vi "Puma_GCS_v2.1_UserVersion.vi"(0 "?":refnum<visa-resource-name>="COM3", 1 "?":u32=9600, 9 "XON":u8=17 format="%.0x", 14 "XOFF":u8=19 format="%.0x", 15 "?":u32=10000, 21 "?":bool=TRUE, 24 "?":u8=10 format="%.0x", 25 "bsize":u32=4096) -> ()   [LabVIEW 2015]
doc: "The Advanced Serial Read and Write example performs a Serial Port Read, a Serial Port Write, or a combination of these actions while setting some advanced serial features like buffer size, termination characters, and XON/XOFF flow control. The user selects the actions (read or write) on the front panel. If both are selected, the VI will write the data first, read the data and then close the VISA session that is opened to the port. \n\nThe parameters set for the serial port must match the parameters of the connected instrument or device. In this example, the bytes to read parameter specifies the number of bytes that the serial port reads. If there were more bytes at the port than the number specified in bytes to read, those bytes would not be read. Also, if you specify to read more bytes than the number of bytes actually read, you might receive a timeout error message.\n\nINSTRUCTIONS:\n1) Select the serial resource and configuration parameters (baud rate, data bits, parity, stop bits, flow control).\n2) Termination character can be enabled and set. Also, set the required input buffer size prior to running the example.\n3) Select the operations to be performed. \n4) Connect the serial port to your device. If no device is available, perform a loopback test by doing one of the following. Short pins 2 and 3 on a RS-232 cable or short pin 4 to pin 8 and pin 5 to pin 9 on a RS-485/422 cable. \n5) Run the VI to see the data read. (The \"read string\" will match the \"string to write\" if a loopback test was performed.)\n\nThis example exposes several advanced features that you may need for your application. Not all applications need all the features shown in this example. The input buffer size is likely an important setting that you want to control in your application. This example expands upon the flow control option for XON and XOFF, allowing the user to choose those control characters. The timeout parameter has been brought to the front panel so a user can specify the time period the VISA Read will wait for the number of bytes to read before timing out. Also, the user has several controls for the termination character, which is discussed later.\n\nNote that you can press the write and read buttons and change the bytes to read parameters on the fly, while the example is running. However, you must stop the example to change the other configuration parameters after the example has started running, and then run again.\n\nSet the I/O buffer size slightly higher the amount of data you expect to receive. This is very important for applications that don't use flow control, as you may lose characters if the receive buffer overflows.\n\nSetting the timeout period ensures that the operation returns with a timeout error if the operation cannot be performed in the specified time period. \n\nSome devices require a termination character in order to identify the end of command strings. Some devices send a termination character to signify the end of data to be read. \n\nThis example shows how you can end the Read operation once a termination character is detected in the buffer and/or append a termination character at the end of the Write data. To enable the Read to end on a termination character, use the VISA Configure Serial Port or use the VISA Properties Serial End Mode for Reads, Termination Character Enable, and Termination Character. To end the Write with a termination character, use the VISA Properties Serial End Mode for Writes, the Send End Enable, and Termination Character. In this example, the same termination character is used for both the Read and the Write. You can specify two different characters for your application, if desired.\n\nYour application may require specific characters for the XON/XOFF Flow Control. You can specify these characters with the VISA Properties Flow Control XOFF Character and Flow Control XON Character. Note that if the standard XON and XOFF characters are used, then decimal 17 and 19 are unavailable for data values. Remember that using flow control and setting an adequate buffer size allow you to prevent buffer overflows."
uses:
  <vilib>/Instr/_visa.llb/VISA Configure Serial Port (Instr).vi
panel:
  in  "Fan Shutdown":bool
  in  "DValve / AV6-T":bool
  in  "Flight Control Board":bool
  in  "Safety":bool
  in  "Test Run":bool
  in  "Reset Control":bool
  in  "Primary Safety 2":bool
  out "?":bool
  out "Motors":cluster{dbl, dbl, dbl, dbl}(graph)={1000.0, 1000.0, 1000.0, 1000.0}
  in  "Pressure Transducers":T1(tab)
  out "?":cluster{dbl, dbl, dbl, dbl, dbl}(graph)
  out "?":cluster{dbl, dbl}(graph)
  in  "Thermocouples":T2(tab)
  out "?":cluster{dbl, dbl, dbl, dbl}(graph)
  out "?":cluster{dbl, dbl}(graph)
  out "fo-u":bool
  out "av5-m":bool
  out "fc-u":bool
  out "PT1-U > 4900 PSI":bool
  out "Takeoff Started":bool
  out "Iterations":i32
  out "Reset Triggered":bool
  in  "PixHawk":bool
  in  "XON 2":u8=17 format="%.0x"
  in  "XOFF 2":u8=19 format="%.0x"
  in  "?":bool=TRUE
  in  "bsize 2":u32=4096
  in  "?":u8=10 format="%.0x"
  in  "?":bool=TRUE
  in  "?":u32=10000
  in  "?":refnum<visa-resource-name>="COM3"
  in  "?":u32=9600
  out "Max Values":T3={20.764332288, 0.0, 0.0, 0.0, 0.0, 0.0, 0.0, 201.058, 25.138999999999953, 0.0, 57.16000000000008, 0.0, 8.920000000000016, 15.403999999999996}
  in  "Data Filename":string
  out "Offset 7":dbl=-251.3
  out "Multiplier 7":dbl=1.264
  out "Offset 6":dbl=-250.2
  out "Offset 5":dbl=-250.3
  out "Offset 4":dbl=-1253.0
  out "Offset 3":dbl=-250.9
  out "Offset 2":dbl=-249.8
  out "Offset 1":dbl=-251.0
  out "Multiplier 6":dbl=1.264
  out "Multiplier 5":dbl=1.277
  out "Multiplier 4":dbl=6.36
  out "Multiplier 3":dbl=1.274
  out "Multiplier 2":dbl=1.267
  out "Multiplier 1":dbl=1.277
  in  "Begin Checklist":bool
  out "Manual Abort Tested":bool
  out "Flight Control On":bool
  out "Reset Triggered 2":bool
  out "Primary Safety Active":bool
  out "Craft Triggered Softkill Active":bool
  out "Hardkill Active":bool
  out "ms":dbl=163640.0
  out "vcc 6":bool
  out "gnd 6":bool=TRUE
  out "TCp-2":bool
  out "vcc 5":bool
  out "gnd 5":bool=TRUE
  out "TCp-1":bool
  out "vcc 4":bool
  out "gnd 4":bool=TRUE
  out "TCpw-4":bool
  out "vcc 3":bool
  out "gnd 3":bool=TRUE
  out "TCpw-3":bool
  out "vcc 2":bool
  out "gnd 2":bool=TRUE
  out "TCpw-2":bool
  out "vcc":bool
  out "gnd":bool=TRUE
  out "TCpw-1":bool
  out "Engine 4":dbl=1000.0
  out "Engine 3":dbl=1000.0
  out "Engine 2":dbl=1000.0
  out "Engine 1":dbl=1000.0
  out "soft kill ind":bool
  out "dump fuel ind":bool
  out "abort ind":bool
  out "run ind":bool
  out "av6-t ind":bool
  out "Control input":bool
  out "return":bool
  out "Control (on/off)":bool
  out "PT5-M":dbl=-6.084000000000003
  out "PT2-M":dbl=-10.039999999999992
  out "PT2-U":dbl=-250.3
  out "PT1-U":dbl=-38.24000000000001
  out "PT3-M":dbl=-141.336
  out "PT1-M":dbl=9.934999999999945
  out "PT4-M":dbl=181.90299999999996
  out "TCp-2":dbl=-2.0
  out "TCp-1":dbl=-2.0
  out "TCpw-4":dbl=-2.0
  out "TCpw-3":dbl=-2.0
  out "TCpw-2":dbl=-2.0
  out "TCpw-1":dbl=-2.0
  out "Output":string="h:;"
  in  "?":enum32{"Test"}(tab)
  in  "Primary Safety":bool=TRUE
  in  "Soft Kill":bool
  in  "Simulate":bool
  in  "Reset FC":bool
  in  "Full Power":bool
  in  "Secondary Safety":bool=TRUE
  in  "Takeoff":bool
  in  "Calibrate":bool
  in  "Profile Selector":u16 max=9 step=1
  in  "abort":bool
  out "?":dbl(graph)=20.40794784
  in  "Send":bool=TRUE
  in  "Recieve":bool=TRUE
  in  "bytes to read 2":u32=1000
  out "?":u32=107
  out "?":string[](array[string])=["339", "205", "86", "191", "0", "190", "194", "-2.00", "-2.00", "-2.00", "-2.00", "-2.00", "-2.00", "555", "1000", "1000", "1000", "1000", "163640"]
  out "?":string[](array[string])=["p:339,205,86,191,0,190,194", "t:-2.00,-2.00,-2.00,-2.00,-2.00,-2.00", "v:555", "m:1000,1000,1000,1000", "h:", "s:163640", ""]
  out "Voltage Sensor":dbl=20.40794784
  in  "dump fuel":bool
  in  "?":enum32{"Ignore"}(tab)
  out "?":bool=TRUE
  out "String":string
  in  "String 3":string
  in  "?":bool=TRUE
  in  "tank iso":bool
  in  "Av-6Tt":bool
  in  "FC-U Toggle":bool
  in  "FOU":bool
  out "?":dbl(slide) scale=0.2..200.0
  out "FO-U":bool
  out "FC-U":bool
  out "AV6-T":bool
  out "AV1-T":bool
  out "AV3-T":bool
  out "AV4-T":bool
  out "AV5-T":bool
  out "AV2-T":bool
  # "Data From Craft:"
  # "FO-U"
  # "FC-U"
  # "receive"
  # "send"
  # "AV6-M"
  # "AV5-M"
  # "AV1-M"
  # "AV2-M"
  # "AV3-M"
  # "AV4-M"
  # "green=open - check thermocouple attachments\nred=short gnd - contact Power or GNC\nblue=short vcc - contact Power or GNC"
  # "Voltage"
  # "TCp2-M"
  # "Tcw1-E"
  # "TCp1-M"
  # "TCw4-E"
  # "TCw3-E"
  # "TCw2-E"
  # "PT4-M"
  # "PT1-M"
  # "PT3-M"
  # "PT1-U"
  # "PT2-U"
  # "PT2-M"
  # "PT5-M"
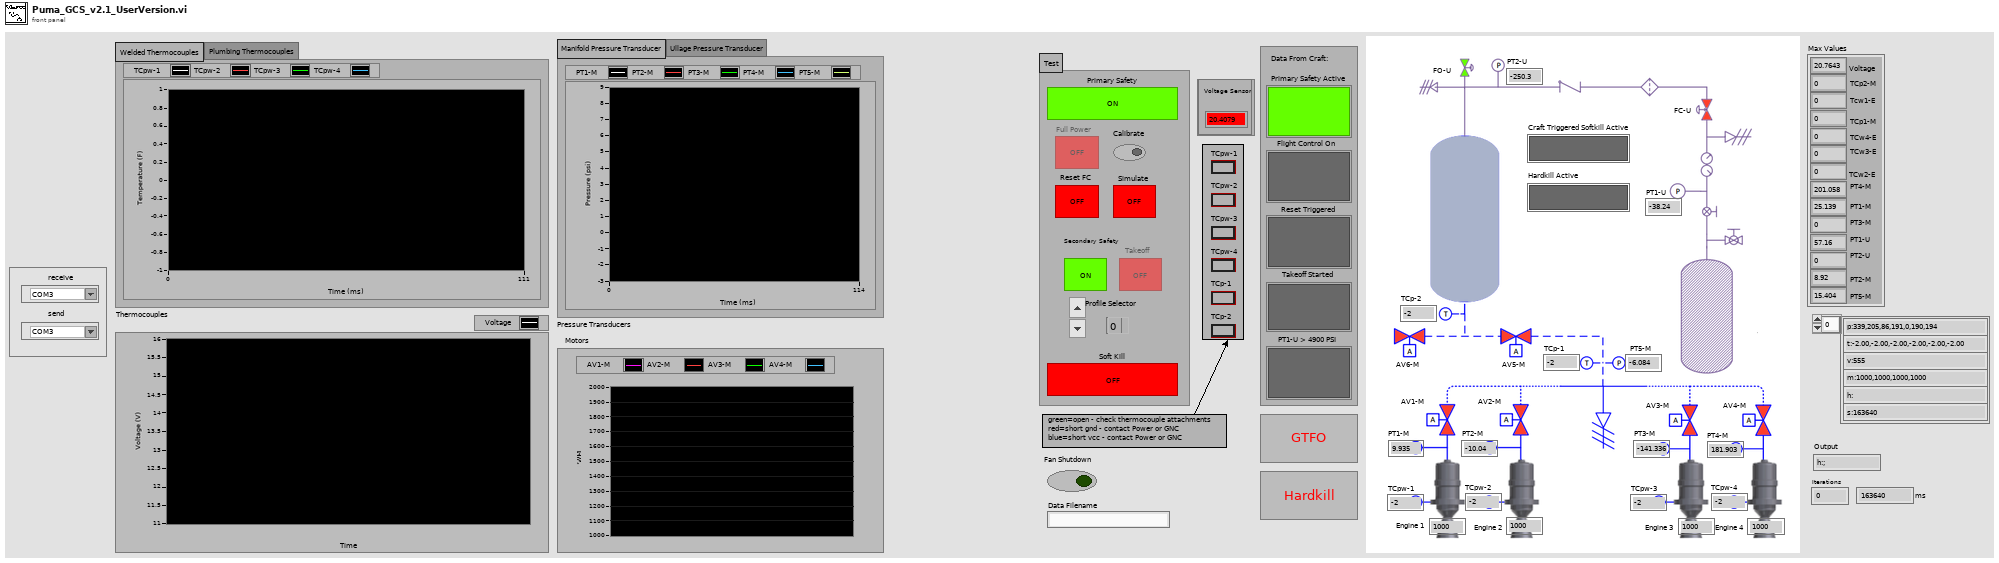
[diagram p1: front panel]
types:
  T1 = enum32{"Manifold Pressure Transducer", "Ullage Pressure Transducer"}
  T2 = enum32{"Welded Thermocouples", "Plumbing Thermocouples"}
  T3 = cluster{dbl, dbl, dbl, dbl, dbl, dbl, dbl, dbl, dbl, dbl, dbl, dbl, dbl, dbl}
  T4 = enum16{"open", "replace", "create", "open or create", "replace or create", "replace or create with confirmation"}
  T5 = cluster{"Output":dbl, dbl, dbl, dbl, dbl, dbl, dbl, "Output":dbl, "Output":dbl, "Output":dbl, "Output":dbl, "Output":dbl, "Output":dbl, "Output":dbl}
  T6 = cluster{"Output":dbl, "Output":dbl, "Output":dbl, "Output":dbl, "Output":dbl}
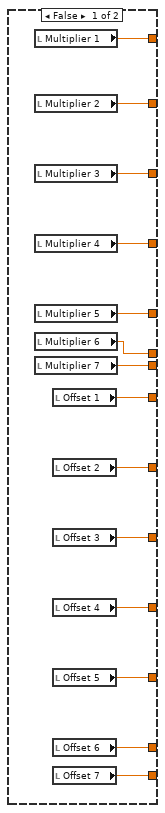
[diagram p3: hidden frame]
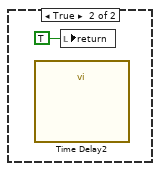
[diagram p13: hidden frame]
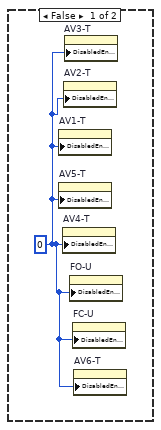
[diagram p16: hidden frame]
diagram:
  w2 = TRUE
  w1 = FALSE
  w51 = u16 16  # I/O Receive Buffer mask
  w75 = u16 16  # I/O Receive Buffer mask
  # "Comment"
  # "Set default values"
  n1 = while {
    stop <- FALSE stop-if-true
    n2 = case shown="True" "Calibrate" {
      tunnel: [w109 w123] -> w93
      tunnel: [w108 w122] -> w92
      tunnel: [w107 w121] -> w91
      tunnel: [w106 w120] -> w90
      tunnel: [w105 w119] -> w89
      tunnel: [w104 w118] -> w88
      tunnel: [w103 w117] -> w87
      tunnel: [w101 w116] -> w86
      tunnel: [w102 w115] -> w85
      tunnel: [w100 w114] -> w84
      tunnel: [w99 w113] -> w83
      tunnel: [w98 w112] -> w82
      tunnel: [w97 w111] -> w81
      tunnel: [w96 w110] -> w80
      frame False {
        n3 = local read "Multiplier 1"() -> (w109:dbl)
        n4 = local read "Multiplier 2"() -> (w108:dbl)
        n5 = local read "Multiplier 3"() -> (w107:dbl)
        n6 = local read "Multiplier 4"() -> (w106:dbl)
        n7 = local read "Multiplier 5"() -> (w105:dbl)
        n8 = local read "Multiplier 6"() -> (w104:dbl)
        n9 = local read "Multiplier 7"() -> (w103:dbl)
        n10 = local read "Offset 1"() -> (w101:dbl)
        n11 = local read "Offset 2"() -> (w102:dbl)
        n12 = local read "Offset 3"() -> (w100:dbl)
        n13 = local read "Offset 4"() -> (w99:dbl)
        n14 = local read "Offset 5"() -> (w98:dbl)
        n15 = local read "Offset 6"() -> (w97:dbl)
        n16 = local read "Offset 7"() -> (w96:dbl)
      }
      frame True {
        n17 = call "P configure.vi"() -> ("Multiplier 1"=w123:dbl, "Offset 1"=w116:dbl, "Multiplier 2"=w122:dbl, "Offset 2"=w115:dbl, "Multiplier 3"=w121:dbl, "Offset 6"=w111:dbl, "Offset 3"=w114:dbl, "Offset 7"=w110:dbl, "Multiplier 4"=w120:dbl, "Multiplier 7"=w117:dbl, "Multiplier 6"=w118:dbl, "Offset 5"=w112:dbl, "Multiplier 5"=w119:dbl, "Offset 4"=w113:dbl)  [unwired: 2 in]
      }
    }
    "Multiplier 1" <- w93
    "Multiplier 2" <- w92
    "Multiplier 3" <- w91
    "Multiplier 4" <- w90
    "Multiplier 5" <- w89
    "Offset 1" <- w86
    "Offset 2" <- w85
    "Offset 3" <- w84
    "Offset 4" <- w83
    "Offset 5" <- w82
    "Offset 6" <- w81
    "Multiplier 7" <- w87
    "Offset 7" <- w80
    "Multiplier 6" <- w88
  }
  n18 = while {
    stop <- FALSE stop-if-true
    n19 = local read "Control (on/off)"() -> (w124:bool)
    n20 = Wait Until Next ms Multiple(millisecond multiple=50) -> ()  [unwired: 1 out]
    n21 = case shown="True" w124 {
      frame False {
      }
      frame True {
        n22 = local read "dump fuel ind"() -> (w142:bool)
        n23 = local read "soft kill ind"() -> (w140:bool)
        n24 = local read "av6-t ind"() -> (w143:bool)
        n25 = local read "abort ind"() -> (w144:bool)
        n26 = local read "fc-u"() -> (w130:bool)
        n27 = local read "av5-m"() -> (w132:bool)
        n28 = local read "fo-u"() -> (w134:bool)
        n29 = local read "run ind"() -> (w141:bool)
        n30 = case shown="True" w140 {
          tunnel: [_ "Are you sure you want to Softkill?"] -> w135
          frame False {
          }
          frame True {
          }
        }
        n31 = case shown="True" w142 {
          tunnel: [_ "Are you sure you want to Dump Fuel?"] -> w137
          frame False {
          }
          frame True {
          }
        }
        n32 = case shown="True" w143 {
          tunnel: [_ "Are you sure you want to Open AV6-M?"] -> w138
          frame False {
          }
          frame True {
          }
        }
        n33 = case shown="True" w144 {
          tunnel: [_ "Are you sure you want to Abort?"] -> w139
          frame False {
          }
          frame True {
          }
        }
        n34 = case shown="True" w134 {
          tunnel: [_ "Are you sure you want to close FO-U?"] -> w133
          frame False {
          }
          frame True {
          }
        }
        n35 = case shown="True" w130 {
          tunnel: [_ "Are you sure you want to open FC-U?"] -> w129
          frame False {
          }
          frame True {
          }
        }
        n36 = case shown="True" w132 {
          tunnel: [_ "Are you sure you want to open AV5-M?"] -> w131
          frame False {
          }
          frame True {
          }
        }
        n37 = case shown="True" w141 {
          tunnel: [_ "Are you sure you want to Run?"] -> w136
          frame False {
          }
          frame True {
          }
        }
        n38 = Concatenate Strings(w135, w136, w137, w138, w139, w133, w131, w129) -> (w128:string)
        n39 = call "DialogBoxSubVI.vi"("Prompt"=w128) -> ("Boolean"=w127:bool)  [unwired: 9 in]
        n40 = case shown="False" w127 {
          frame False {
            n41 = call "Time Delay"() -> ()  [unwired: 11 in, 1 out]
            n42 = local write "return"(TRUE) -> ()
          }
          frame True {
            n43 = call "Time Delay2"() -> ()  [unwired: 11 in, 1 out]
            n44 = local write "return"(TRUE) -> ()
          }
        }
        n45 = local write "Control input"(w127) -> ()
      }
    }
  }
  n46 = call-poly "VISA Configure Serial Port"("VISA resource name"="?", "timeout (10sec)"="?", "termination char\n(0xA = '\\n' = LF)"="?", "Enable Termination\nChar (T)"="?", "baud rate (9600)"="?") -> ("VISA resource name out"=w64:refnum<visa-resource-name>, "error out"=w67:errorcluster)  [unwired: 5 in, 4 out]
  n47 = call-poly "VISA Configure Serial Port"("VISA resource name"="?", "timeout (10sec)"="?", "termination char\n(0xA = '\\n' = LF)"="?", "Enable Termination\nChar (T)"="?", "baud rate (9600)"="?") -> ("VISA resource name out"=w40:refnum<visa-resource-name>, "error out"=w43:errorcluster)  [unwired: 5 in, 4 out]
  n48 = case shown="True" "?" {
    selector: "?" -> [_ w157]
    tunnel: w64 -> [w155 w163]
    tunnel: w67 -> [w156 w162]
    tunnel: [w155 w161] -> w65
    tunnel: [w156 w160] -> w66
    tunnel: "?" -> [_ w158]
    frame False {
    }
    frame True {
      w159 = u16 2 items=["None", "LastBit", "TermChar", "Break"] ("Serial Settings:Serial End Mode for Writes")
      n49 = property class="Instr"(reference=w163, error in=w162, "Serial Settings:End Mode for Writes"=w159, "Message Based Settings:Send End Enable"=w157, "Message Based Settings:Termination Character"=w158) -> (reference out=w161:refnum<visa-resource-name>, error out=w160:errorcluster)
    }
  }
  n50 = case shown="True" "?" {
    selector: "?" -> [_ w166]
    tunnel: w40 -> [w164 w172]
    tunnel: w43 -> [w165 w171]
    tunnel: [w164 w170] -> w41
    tunnel: [w165 w169] -> w42
    tunnel: "?" -> [_ w167]
    frame False {
    }
    frame True {
      w168 = u16 2 items=["None", "LastBit", "TermChar", "Break"] ("Serial Settings:Serial End Mode for Writes")
      n51 = property class="Instr"(reference=w172, error in=w171, "Serial Settings:End Mode for Writes"=w168, "Message Based Settings:Send End Enable"=w166, "Message Based Settings:Termination Character"=w167) -> (reference out=w170:refnum<visa-resource-name>, error out=w169:errorcluster)
    }
  }
  n52 = property on="Secondary Safety" class="Bool (strict)"("Value"=w2) -> ()  [unwired: 2 in, 2 out]
  n53 = property on="Primary Safety" class="Bool (strict)"("Value"=w2) -> ()  [unwired: 2 in, 2 out]
  n54 = property on="Reset FC" class="Bool (strict)"("Value"=w1) -> ()  [unwired: 2 in, 2 out]
  n55 = property on="Simulate" class="Bool (strict)"("Value"=w1) -> ()  [unwired: 2 in, 2 out]
  n56 = property on="Craft Triggered Softkill Active" class="Bool (strict)"("Value"=w1) -> ()  [unwired: 2 in, 2 out]
  n57 = property on="Hardkill Active" class="Bool (strict)"("Value"=w1) -> ()  [unwired: 2 in, 2 out]
  n58 = property on="Takeoff Started" class="Bool (strict)"("Value"=w1) -> ()  [unwired: 2 in, 2 out]
  n59 = property on="FOU" class="Bool (strict)"("Value"=w1) -> ()  [unwired: 2 in, 2 out]
  n60 = property on="Soft Kill" class="Bool (strict)"("Value"=w1) -> ()  [unwired: 2 in, 2 out]
  n61 = property on="dump fuel" class="Bool (strict)"("Value"=w1) -> ()  [unwired: 2 in, 2 out]
  n62 = property on="abort" class="Bool (strict)"("Value"=w1) -> ()  [unwired: 2 in, 2 out]
  n63 = property on="Manual Abort Tested" class="Bool (strict)"("Value"=w1) -> ()  [unwired: 2 in, 2 out]
  n64 = Build Path(base path=path "C:/Users/Lunar Lion/Desktop/Puma_Test_Data" ("file path (use dialog)"), name or relative path="Data Filename") -> (appended path=w59:path)
  n65 = Build Array("PT4-M_a", "PT1-M_a", "PT3-M_a", "PT1-U_a", "PT2-U_a", "PT2-M_a", "PT5-M_a", "PT4-M", "PT1-M", "PT3-M", "PT1-U", "PT2-U", "PT2-M", "PT5-M", "TCp2-M", "TCw1-E", "TCp1-M", "TCw4-E", "TCw3-E", "TCw2-E", "Voltage", "Motor1", "Motor2", "Motor3", "Motor4", "Statestring") -> (w12:string[])
  n66 = VISA Set I/O Buffer Size(VISA resource name=w65, mask (16)=w75, size (4096)="bsize", error in (no error)=w66) -> (VISA resource name out=w71:refnum<visa-resource-name>, error out=w70:errorcluster)
  n67 = VISA Set I/O Buffer Size(VISA resource name=w41, mask (16)=w51, size (4096)="bsize 2", error in (no error)=w42) -> (VISA resource name out=w47:refnum<visa-resource-name>, error out=w46:errorcluster)
  n68 = Open/Create/Replace File(file path (use dialog)=w59, operation (0:open)=T4."replace or create with confirmation") -> (refnum out=w9:refnum<file>)  [unwired: 4 in, 2 out]
  n69 = Array To Spreadsheet String(array=w12, 3:"%s" ("format string")) -> (spreadsheet string=w10:string)  [unwired: 1 in]
  n70 = property class="Instr"(reference=w71, error in=w70, "Serial Settings:Flow Control XON Character"="XON", "Serial Settings:Flow Control XOFF Character"="XOFF") -> (reference out=w63:refnum<visa-resource-name>, error out=w62:errorcluster)
  n71 = property class="Instr"(reference=w47, error in=w46, "Serial Settings:Flow Control XON Character"="XON 2", "Serial Settings:Flow Control XOFF Character"="XOFF 2") -> (reference out=w39:refnum<visa-resource-name>)  [unwired: 1 out]
  n72 = Write to Text File(file (use dialog)=w9, text=w10) -> (refnum out=w8:refnum<file>)  [unwired: 2 in, 2 out]
  n73 = while {
    tunnel: w63 -> [w338]
    tunnel: w62 -> [w406]
    tunnel: [w322] -> w7
    tunnel: [w321] -> w61
    shift-right: [w506] -> _
    shift-left: _ -> [w505]
    shift-right: [w231] -> _
    shift-left: _ -> [w467]
    shift-right: [w475] -> _
    shift-left: _ -> [w476]
    shift-right: [w466] -> _
    shift-left: _ -> [w490]
    shift-right: [w249] -> _
    shift-left: _ -> [w488]
    shift-right: [w468] -> _
    shift-left: _ -> [w471]
    shift-right: ["Begin Checklist"] -> _
    shift-left: _ -> [w387]
    tunnel: w8 -> [w359]
    tunnel: [w356] -> w58
    shift-right: [w341] -> _
    shift-left: T3 {0.0, 0.0, 0.0, 0.0, 0.0, 0.0, 0.0, 0.0, 0.0, 0.0, 0.0, 0.0, 0.0, 0.0} -> [w340]
    tunnel: w39 -> [_]
    shift-right: [w245] -> _
    shift-left: _ -> [w248]
    shift-right: [w242] -> _
    shift-left: _ -> [w243]
    shift-right: [w239] -> _
    shift-left: _ -> [w240]
    i -> [w326]
    stop <- FALSE stop-if-true
    w193 = 140.0
    w195 = 1400.0
    w200 = 900.0
    w270 = u32 13816530
    w272 = 120.0
    w275 = 1200.0
    w271 = u32 16776704
    w281 = 800.0
    # "e"
    # "The purpose of this indicator is not entirely clear"
    # "Hidden test run button."
    # "Hidden secondary safety."
    # "Hidden reset control button."
    # "Hidden flight control board button."
    # "Un-named indicator, hidden."
    # "Hidden dump valve indicator/button?"
    # "Hidden primary safety"
    # "Tabs for the main command buttons."
    # "Ignore tab with the two strings and indicator light."
    # "Above nominal thresholds:\n   All PTs except PT1-U: 800\n   TCpw-1 to 4: 1200\n   TCp-1 and 2: 120"
    # "The second String \nParsing Indicator"
    # "String Parsing Indicator control"
    # "ENSURE THE PTs ARE HOOKED UP PROPERLY"
    # "Here, if PT1-U indicates a pressure greater than 5000 psi,\nthe indicator represented in the case structure is turned green. Otherwise, it is turned red."
    # "AV6 -T Case"
    # "AV5-T Case"
    # "AV5-T Toggle"
    n74 = case shown="True" FALSE {
      frame False {
      }
      frame True {
        w678 = FALSE
        n75 = local write "FOU"(TRUE) -> ()
        n76 = local write "AV1-T"(w678) -> ()
        n77 = local write "AV2-T"(w678) -> ()
        n78 = local write "AV3-T"(w678) -> ()
        n79 = local write "AV4-T"(w678) -> ()
        n80 = local write "FC-U Toggle"(w678) -> ()
        n81 = local write "tank iso"(w678) -> ()
      }
    }
    n82 = property on="abort" class="Bool (strict)"() -> ("Value"=w302:bool)  [unwired: 2 in, 2 out]
    n83 = local read "Voltage Sensor"() -> (w234:dbl)
    n84 = case shown="False" w302 {
      frame False {
        n85 = property on="Soft Kill" class="Bool (strict)"() -> ("Value"=w661:bool)  [unwired: 2 in, 2 out]
        n86 = case shown="True" w661 {
          frame False {
            n87 = property on="dump fuel" class="Bool (strict)"("DisabledEnum"=0) -> ()  [unwired: 2 in, 2 out]
          }
          frame True {
            n88 = property on="dump fuel" class="Bool (strict)"("DisabledEnum"=2) -> ()  [unwired: 2 in, 2 out]
          }
        }
      }
      frame True {
        n89 = property on="dump fuel" class="Bool (strict)"("DisabledEnum"=2) -> ()  [unwired: 2 in, 2 out]
      }
    }
    n90 = Greater?(x=w234, y=14.5) -> (0:w237:bool)
    n91 = Less Or Equal?(x=w234, y=16.8) -> (x <= y?=w317:bool)
    n92 = Less Or Equal?(x=w234, y=15.5) -> (x <= y?=w312:bool)
    n93 = Greater?(x=w234, y=15.5) -> (0:w316:bool)
    n94 = Greater?(x=w234, y=16.8) -> (0:w309:bool)
    n95 = Less Or Equal?(x=w234, y=17.0) -> (x <= y?=w310:bool)
    n96 = Greater?(x=w234, y=17.0) -> (0:w305:bool)
    n97 = And(x=w309, y=w310) -> (x .and. y?=w308:bool)
    n98 = And(x=w237, y=w312) -> (x .and. y?=w313:bool)
    n99 = And(x=w316, y=w317) -> (x .and. y?=w318:bool)
    n100 = Less Or Equal?(x=w234, y=14.5) -> (x <= y?=w235:bool)
    n101 = case shown="True" w313 {
      frame False {
      }
      frame True {
        n102 = property on="Voltage Sensor" class="DigNum (strict)"("NumText.TextColor"=u32 0) -> ()  [unwired: 2 in, 2 out]
        n103 = property on="Voltage Sensor" class="DigNum (strict)"("NumText.BGColor"=u32 16776704) -> ()  [unwired: 2 in, 2 out]
      }
    }
    n104 = case shown="True" w235 {
      frame False {
      }
      frame True {
        n105 = property on="Voltage Sensor" class="DigNum (strict)"("NumText.BG Color"=u32 16711680) -> ()  [unwired: 2 in, 2 out]
      }
    }
    n106 = case shown="True" w318 {
      frame False {
      }
      frame True {
        n107 = property on="Voltage Sensor" class="DigNum (strict)"("NumText.BGColor"=u32 6618880) -> ()  [unwired: 2 in, 2 out]
        n108 = property on="Voltage Sensor" class="DigNum (strict)"("NumText.TextColor"=u32 16777222) -> ()  [unwired: 2 in, 2 out]
      }
    }
    n109 = case shown="True" w308 {
      frame False {
      }
      frame True {
        n110 = property on="Voltage Sensor" class="DigNum (strict)"("NumText.BGColor"=u32 16776704) -> ()  [unwired: 2 in, 2 out]
        n111 = property on="Voltage Sensor" class="DigNum (strict)"("NumText.TextColor"=u32 16777222) -> ()  [unwired: 2 in, 2 out]
      }
    }
    n112 = case shown="True" w305 {
      frame False {
      }
      frame True {
        n113 = property on="Voltage Sensor" class="DigNum (strict)"("NumText.BGColor"=u32 16711704) -> ()  [unwired: 2 in, 2 out]
      }
    }
    n114 = Exclusive Or(1:w490, 2:"abort") -> (0:w492:bool)
    n115 = property on="TCpw-1" class="DigNum (strict)"() -> ("Value"=w196:dbl)  [unwired: 2 in, 2 out]
    n116 = property on="TCpw-2" class="DigNum (strict)"() -> ("Value"=w197:dbl)  [unwired: 2 in, 2 out]
    n117 = property on="TCpw-3" class="DigNum (strict)"() -> ("Value"=w198:dbl)  [unwired: 2 in, 2 out]
    n118 = property on="TCpw-4" class="DigNum (strict)"() -> ("Value"=w199:dbl)  [unwired: 2 in, 2 out]
    n119 = case shown="True" w492 {
      tunnel: [w742 w744] -> w466
      tunnel: w490 -> [w742 w743]
      frame False {
      }
      frame True {
        n120 = case shown="False" w743 {
          tunnel: [w745 FALSE ("T button?")] -> w744
          frame False {
            w746 = TRUE
            n121 = local write "abort ind"(w746) -> ()
            n122 = local write "Control (on/off)"(w746) -> ()
            n123 = local read "Control input"() -> (w745:bool)
          }
          frame True {
          }
        }
      }
    }
    n124 = Exclusive Or(1:w471, 2:"Soft Kill") -> (0:w469:bool)
    n125 = property on="TCp-2" class="DigNum (strict)"() -> ("Value"=w192:dbl)  [unwired: 2 in, 2 out]
    n126 = property on="TCp-1" class="DigNum (strict)"() -> ("Value"=w194:dbl)  [unwired: 2 in, 2 out]
    n127 = property on="PT2-M" class="DigNum (strict)"() -> ("Value"=w201:dbl)  [unwired: 2 in, 2 out]
    n128 = property on="PT1-M" class="DigNum (strict)"() -> ("Value"=w202:dbl)  [unwired: 2 in, 2 out]
    n129 = property on="PT3-M" class="DigNum (strict)"() -> ("Value"=w203:dbl)  [unwired: 2 in, 2 out]
    n130 = property on="PT4-M" class="DigNum (strict)"() -> ("Value"=w204:dbl)  [unwired: 2 in, 2 out]
    n131 = property on="PT5-M" class="DigNum (strict)"() -> ("Value"=w205:dbl)  [unwired: 2 in, 2 out]
    n132 = property on="PT2-U" class="DigNum (strict)"() -> ("Value"=w206:dbl)  [unwired: 2 in, 2 out]
    n133 = Exclusive Or(1:w488, 2:"dump fuel") -> (0:w489:bool)
    n134 = case shown="True" w469 {
      tunnel: [w732 w734] -> w468
      tunnel: w471 -> [w732 w733]
      frame False {
      }
      frame True {
        n135 = case shown="False" w733 {
          tunnel: [w735 _] -> w734
          frame False {
            w736 = TRUE
            n136 = local write "soft kill ind"(w736) -> ()
            n137 = local write "Control (on/off)"(w736) -> ()
            n138 = local read "Control input"() -> (w735:bool)
          }
          frame True {
          }
        }
      }
    }
    n139 = Greater Or Equal?(x=w192, y=w272) -> (x >= y?=w273:bool)
    n140 = Greater Or Equal?(x=w194, y=w272) -> (x >= y?=w274:bool)
    n141 = Greater Or Equal?(x=w196, y=w275) -> (x >= y?=w279:bool)
    n142 = Greater Or Equal?(x=w197, y=w275) -> (x >= y?=w278:bool)
    n143 = Greater Or Equal?(x=w198, y=w275) -> (x >= y?=w277:bool)
    n144 = Greater Or Equal?(x=w199, y=w275) -> (x >= y?=w276:bool)
    n145 = Greater Or Equal?(x=w201, y=w281) -> (x >= y?=w285:bool)
    n146 = Greater Or Equal?(x=w202, y=w281) -> (x >= y?=w286:bool)
    n147 = Greater Or Equal?(x=w203, y=w281) -> (x >= y?=w284:bool)
    n148 = Greater Or Equal?(x=w204, y=w281) -> (x >= y?=w283:bool)
    n149 = Greater Or Equal?(x=w205, y=w281) -> (x >= y?=w282:bool)
    n150 = Greater Or Equal?(x=w206, y=w281) -> (x >= y?=w280:bool)
    n151 = case shown="True" w489 {
      tunnel: [w737 w739] -> w249
      tunnel: w488 -> [w737 w738]
      frame False {
      }
      frame True {
        n152 = case shown="False" w738 {
          tunnel: [w741 _] -> w739
          frame False {
            w740 = TRUE
            n153 = local write "Control (on/off)"(w740) -> ()
            n154 = local write "dump fuel ind"(w740) -> ()
            n155 = local read "Control input"() -> (w741:bool)
          }
          frame True {
          }
        }
      }
    }
    n156 = case shown="True" w273 {
      tunnel: w271 -> [_ w593]
      tunnel: w270 -> [w589 _]
      tunnel: w193 -> [_ w591]
      tunnel: w192 -> [_ w590]
      frame False {
        n157 = property on="TCp-2" class="DigNum (strict)"("NumText.BGColor"=w589) -> ()  [unwired: 2 in, 2 out]
      }
      frame True {
        n158 = Greater Or Equal?(x=w590, y=w591) -> (x >= y?=w592:bool)
        n159 = property on="TCp-2" class="DigNum (strict)"("NumText.BGColor"=w593) -> ()  [unwired: 2 in, 2 out]
        n160 = case shown="True" w592 {
          frame False {
          }
          frame True {
            n161 = property on="TCp-2" class="DigNum (strict)"("NumText.BGColor"=u32 16711680) -> ()  [unwired: 2 in, 2 out]
          }
        }
      }
    }
    n162 = case shown="True" w274 {
      tunnel: w271 -> [_ w599]
      tunnel: w270 -> [w595 _]
      tunnel: w194 -> [_ w597]
      tunnel: w193 -> [_ w596]
      frame False {
        n163 = property on="TCp-1" class="DigNum (strict)"("NumText.BGColor"=w595) -> ()  [unwired: 2 in, 2 out]
      }
      frame True {
        n164 = Greater Or Equal?(x=w597, y=w596) -> (x >= y?=w598:bool)
        n165 = property on="TCp-1" class="DigNum (strict)"("NumText.BGColor"=w599) -> ()  [unwired: 2 in, 2 out]
        n166 = case shown="True" w598 {
          frame False {
          }
          frame True {
            n167 = property on="TCp-1" class="DigNum (strict)"("NumText.BGColor"=u32 16711680) -> ()  [unwired: 2 in, 2 out]
          }
        }
      }
    }
    n168 = case shown="True" w279 {
      tunnel: w271 -> [_ w623]
      tunnel: w270 -> [w619 _]
      tunnel: w196 -> [_ w621]
      tunnel: w195 -> [_ w620]
      frame False {
        n169 = property on="TCpw-1" class="DigNum (strict)"("NumText.BGColor"=w619) -> ()  [unwired: 2 in, 2 out]
      }
      frame True {
        n170 = Greater Or Equal?(x=w621, y=w620) -> (x >= y?=w622:bool)
        n171 = property on="TCpw-1" class="DigNum (strict)"("NumText.BGColor"=w623) -> ()  [unwired: 2 in, 2 out]
        n172 = case shown="True" w622 {
          frame False {
          }
          frame True {
            n173 = property on="TCpw-1" class="DigNum (strict)"("NumText.BGColor"=u32 16711680) -> ()  [unwired: 2 in, 2 out]
          }
        }
      }
    }
    n174 = case shown="True" w278 {
      tunnel: w271 -> [_ w617]
      tunnel: w270 -> [w613 _]
      tunnel: w197 -> [_ w615]
      tunnel: w195 -> [_ w614]
      frame False {
        n175 = property on="TCpw-2" class="DigNum (strict)"("NumText.BGColor"=w613) -> ()  [unwired: 2 in, 2 out]
      }
      frame True {
        n176 = Greater Or Equal?(x=w615, y=w614) -> (x >= y?=w616:bool)
        n177 = property on="TCpw-2" class="DigNum (strict)"("NumText.BGColor"=w617) -> ()  [unwired: 2 in, 2 out]
        n178 = case shown="True" w616 {
          frame False {
          }
          frame True {
            n179 = property on="TCpw-2" class="DigNum (strict)"("NumText.BGColor"=u32 16711680) -> ()  [unwired: 2 in, 2 out]
          }
        }
      }
    }
    n180 = case shown="True" w277 {
      tunnel: w271 -> [_ w611]
      tunnel: w270 -> [w607 _]
      tunnel: w198 -> [_ w609]
      tunnel: w195 -> [_ w608]
      frame False {
        n181 = property on="TCpw-3" class="DigNum (strict)"("NumText.BGColor"=w607) -> ()  [unwired: 2 in, 2 out]
      }
      frame True {
        n182 = Greater Or Equal?(x=w609, y=w608) -> (x >= y?=w610:bool)
        n183 = property on="TCpw-3" class="DigNum (strict)"("NumText.BGColor"=w611) -> ()  [unwired: 2 in, 2 out]
        n184 = case shown="True" w610 {
          frame False {
          }
          frame True {
            n185 = property on="TCpw-3" class="DigNum (strict)"("NumText.BGColor"=u32 16711680) -> ()  [unwired: 2 in, 2 out]
          }
        }
      }
    }
    n186 = case shown="True" w276 {
      tunnel: w271 -> [_ w605]
      tunnel: w270 -> [w601 _]
      tunnel: w199 -> [_ w603]
      tunnel: w195 -> [_ w602]
      frame False {
        n187 = property on="TCpw-4" class="DigNum (strict)"("NumText.BGColor"=w601) -> ()  [unwired: 2 in, 2 out]
      }
      frame True {
        n188 = Greater Or Equal?(x=w603, y=w602) -> (x >= y?=w604:bool)
        n189 = property on="TCpw-4" class="DigNum (strict)"("NumText.BGColor"=w605) -> ()  [unwired: 2 in, 2 out]
        n190 = case shown="True" w604 {
          frame False {
          }
          frame True {
            n191 = property on="TCpw-4" class="DigNum (strict)"("NumText.BGColor"=u32 16711680) -> ()  [unwired: 2 in, 2 out]
          }
        }
      }
    }
    n192 = case shown="True" w285 {
      tunnel: w271 -> [_ w653]
      tunnel: w270 -> [w649 _]
      tunnel: w201 -> [_ w651]
      tunnel: w200 -> [_ w650]
      frame False {
        n193 = property on="PT2-M" class="DigNum (strict)"("NumText.BGColor"=w649) -> ()  [unwired: 2 in, 2 out]
      }
      frame True {
        n194 = Greater Or Equal?(x=w651, y=w650) -> (x >= y?=w652:bool)
        n195 = property on="PT2-M" class="DigNum (strict)"("NumText.BGColor"=w653) -> ()  [unwired: 2 in, 2 out]
        n196 = case shown="True" w652 {
          frame False {
          }
          frame True {
            n197 = property on="PT1-M" class="DigNum (strict)"("NumText.BGColor"=u32 16711680) -> ()  [unwired: 2 in, 2 out]
          }
        }
      }
    }
    n198 = case shown="True" w286 {
      tunnel: w271 -> [_ w659]
      tunnel: w270 -> [w655 _]
      tunnel: w202 -> [_ w657]
      tunnel: w200 -> [_ w656]
      frame False {
        n199 = property on="PT1-M" class="DigNum (strict)"("NumText.BGColor"=w655) -> ()  [unwired: 2 in, 2 out]
      }
      frame True {
        n200 = Greater Or Equal?(x=w657, y=w656) -> (x >= y?=w658:bool)
        n201 = property on="PT1-M" class="DigNum (strict)"("NumText.BGColor"=w659) -> ()  [unwired: 2 in, 2 out]
        n202 = case shown="True" w658 {
          frame False {
          }
          frame True {
            n203 = property on="PT1-M" class="DigNum (strict)"("NumText.BGColor"=u32 16711680) -> ()  [unwired: 2 in, 2 out]
          }
        }
      }
    }
    n204 = case shown="True" w284 {
      tunnel: w271 -> [_ w647]
      tunnel: w270 -> [w643 _]
      tunnel: w200 -> [_ w645]
      tunnel: w203 -> [_ w644]
      frame False {
        n205 = property on="PT3-M" class="DigNum (strict)"("NumText.BGColor"=w643) -> ()  [unwired: 2 in, 2 out]
      }
      frame True {
        n206 = Greater Or Equal?(x=w644, y=w645) -> (x >= y?=w646:bool)
        n207 = property on="PT3-M" class="DigNum (strict)"("NumText.BGColor"=w647) -> ()  [unwired: 2 in, 2 out]
        n208 = case shown="True" w646 {
          frame False {
          }
          frame True {
            n209 = property on="PT3-M" class="DigNum (strict)"("NumText.BGColor"=u32 16711680) -> ()  [unwired: 2 in, 2 out]
          }
        }
      }
    }
    n210 = case shown="True" w283 {
      tunnel: w271 -> [_ w641]
      tunnel: w270 -> [w637 _]
      tunnel: w204 -> [_ w639]
      tunnel: w200 -> [_ w638]
      frame False {
        n211 = property on="PT4-M" class="DigNum (strict)"("NumText.BGColor"=w637) -> ()  [unwired: 2 in, 2 out]
      }
      frame True {
        n212 = Greater Or Equal?(x=w639, y=w638) -> (x >= y?=w640:bool)
        n213 = property on="PT4-M" class="DigNum (strict)"("NumText.BGColor"=w641) -> ()  [unwired: 2 in, 2 out]
        n214 = case shown="True" w640 {
          frame False {
          }
          frame True {
            n215 = property on="PT4-M" class="DigNum (strict)"("NumText.BGColor"=u32 16711680) -> ()  [unwired: 2 in, 2 out]
          }
        }
      }
    }
    n216 = case shown="True" w282 {
      tunnel: w271 -> [_ w635]
      tunnel: w270 -> [w631 _]
      tunnel: w205 -> [_ w633]
      tunnel: w200 -> [_ w632]
      frame False {
        n217 = property on="PT5-M" class="DigNum (strict)"("NumText.BGColor"=w631) -> ()  [unwired: 2 in, 2 out]
      }
      frame True {
        n218 = Greater Or Equal?(x=w633, y=w632) -> (x >= y?=w634:bool)
        n219 = property on="PT5-M" class="DigNum (strict)"("NumText.BGColor"=w635) -> ()  [unwired: 2 in, 2 out]
        n220 = case shown="True" w634 {
          frame False {
          }
          frame True {
            n221 = property on="PT5-M" class="DigNum (strict)"("NumText.BGColor"=u32 16711680) -> ()  [unwired: 2 in, 2 out]
          }
        }
      }
    }
    n222 = case shown="True" w280 {
      tunnel: w271 -> [_ w629]
      tunnel: w270 -> [w625 _]
      tunnel: w200 -> [_ w627]
      tunnel: w206 -> [_ w626]
      frame False {
        n223 = property on="PT2-U" class="DigNum (strict)"("NumText.BGColor"=w625) -> ()  [unwired: 2 in, 2 out]
      }
      frame True {
        n224 = Greater Or Equal?(x=w626, y=w627) -> (x >= y?=w628:bool)
        n225 = property on="PT2-U" class="DigNum (strict)"("NumText.BGColor"=w629) -> ()  [unwired: 2 in, 2 out]
        n226 = case shown="True" w628 {
          frame False {
          }
          frame True {
            n227 = property on="PT2-U" class="DigNum (strict)"("NumText.BGColor"=u32 16711680) -> ()  [unwired: 2 in, 2 out]
          }
        }
      }
    }
    n228 = Not(x="Secondary Safety") -> (.not. x?=w327:bool)
    n229 = And(x="Safety", y="Test Run") -> (x .and. y?=w521:bool)
    n230 = And(x=w327, y="Takeoff") -> (x .and. y?=w520:bool)
    n231 = Not(x="Secondary Safety") -> (.not. x?=w329:bool)
    n232 = case shown="False" w329 {
      tunnel: [2 0] -> w328
      frame False {
      }
      frame True {
      }
    }
    n233 = Or(x=w520, y=w521) -> (x .or. y?=w495:bool)
    n234 = case shown="True" "Recieve" {
      tunnel: w406 -> [w799 w804]
      tunnel: w338 -> [w800 w803]
      tunnel: [w799 w806] -> w321
      tunnel: [w800 w805] -> w322
      tunnel: [_ w802] -> _
      tunnel: [_ w801] -> w358
      frame False {
      }
      frame True {
        n235 = case "Read bytes from port." shown="No Error" w804 {
          selector: w804 -> [w809 w815]
          tunnel: [w812 w815] -> w806
          tunnel: [w813 w814] -> w805
          tunnel: w803 -> [w810 w814]
          tunnel: [w807 _] -> w802
          tunnel: [w807 _] -> w801
          frame No Error {
            n236 = VISA Read(VISA resource name=w810, byte count="bytes to read 2", error in (no error)=w809) -> (VISA resource name out=w813:refnum<visa-resource-name>, read buffer=w807:string, return count=→"?":u32, error out=w812:errorcluster)
          }
          frame Error {
          }
        }
      }
    }
    n237 = Exclusive Or(1:w467, 2:w495) -> (0:w494:bool)
    n238 = case shown="True" w494 {
      tunnel: [w748 w750] -> w231
      tunnel: w467 -> [w748 w749]
      frame False {
      }
      frame True {
        n239 = case shown="True" w749 {
          tunnel: [w752 _] -> w750
          frame False {
            w751 = TRUE
            n240 = local write "run ind"(w751) -> ()
            n241 = local write "Control (on/off)"(w751) -> ()
            n242 = local read "Control input"() -> (w752:bool)
          }
          frame True {
            w753 = FALSE
            n243 = local write "Test Run"(w753) -> ()
            n244 = local write "Control (on/off)"(w753) -> ()
            n245 = local write "Takeoff"(w753) -> ()
          }
        }
      }
    }
    "AV1-T" <- w231
    "AV4-T" <- w231
    "AV2-T" <- w231
    "AV3-T" <- w231
    n246 = case shown="True" "tank iso" {
      tunnel: [w577 w579] -> w242
      tunnel: w243 -> [w577 w578]
      frame False {
      }
      frame True {
        n247 = case shown="True" w578 {
          tunnel: [w580 _] -> w579
          frame False {
            w581 = TRUE
            n248 = local write "av5-m"(w581) -> ()
            n249 = local write "Control (on/off)"(w581) -> ()
            n250 = local read "Control input"() -> (w580:bool)
          }
          frame True {
            n251 = local write "tank iso"(FALSE) -> ()
          }
        }
      }
    }
    "AV5-T" <- w242
    n252 = property on="Takeoff" class="Bool (strict)"("DisabledEnum"=w328) -> ()  [unwired: 2 in, 2 out]
    n253 = case shown="True" "FOU" {
      tunnel: [w583 w585] -> w245
      tunnel: w248 -> [w583 w584]
      frame False {
      }
      frame True {
        n254 = case shown="True" w584 {
          tunnel: [w586 _] -> w585
          frame False {
            w587 = TRUE
            n255 = local write "Control (on/off)"(w587) -> ()
            n256 = local read "Control input"() -> (w586:bool)
            n257 = local write "fo-u"(w587) -> ()
          }
          frame True {
            n258 = local write "FOU"(FALSE) -> ()
          }
        }
      }
    }
    "FO-U" <- w245
    n259 = case shown="True" "FC-U Toggle" {
      tunnel: [w571 w573] -> w239
      tunnel: w240 -> [w571 w572]
      frame False {
      }
      frame True {
        n260 = case shown="False" w572 {
          tunnel: [w574 _] -> w573
          frame False {
            w575 = TRUE
            n261 = local write "Control (on/off)"(w575) -> ()
            n262 = local write "fc-u"(w575) -> ()
            n263 = local read "Control input"() -> (w574:bool)
          }
          frame True {
            n264 = local write "FC-U Toggle"(FALSE) -> ()
          }
        }
      }
    }
    "FC-U" <- w239
    n265 = Or(x=w466, y=w468) -> (x .or. y?=w493:bool)
    n266 = Greater?(x="Profile Selector", y=9) -> (0:w187:bool)
    n267 = Less?(x="Profile Selector", y=0) -> (x < y?=w186:bool)
    n268 = Or(x=w493, y=w249) -> (x .or. y?=w463:bool)
    n269 = Or(x=w187, y=w186) -> (x .or. y?=w188:bool)
    n270 = Not(x=w463) -> (.not. x?=w304:bool)
    n271 = case shown="True" w188 {
      frame False {
      }
      frame True {
        n272 = property on="Profile Selector" class="DigNum (strict)"("Value"=0) -> ()  [unwired: 2 in, 2 out]
      }
    }
    n273 = And(x=w304, y="Safety") -> (x .and. y?=w480:bool)
    n274 = And(x=w304, y="Test Run") -> (x .and. y?=w477:bool)
    n275 = And(x=w304, y="Secondary Safety") -> (x .and. y?=w479:bool)
    n276 = And(x=w304, y="Takeoff") -> (x .and. y?=w478:bool)
    n277 = local write "Safety"(w480) -> ()
    n278 = local write "Test Run"(w477) -> ()
    n279 = local write "Takeoff"(w478) -> ()
    n280 = Concatenate Strings(w358, "\n" ("string")) -> ()  [unwired: 1 out]
    n281 = Or(x=w480, y=w479) -> (x .or. y?=w483:bool)
    n282 = Or(x=w478, y=w477) -> (x .or. y?=w482:bool)
    n283 = Spreadsheet String To Array(delimiter (Tab)=";", format string="%d", spreadsheet string=w358, array type (2D Dbl)=string[] ["p:1234.1234.1234.1234,1234,1234", "t:1234,1234,1234"] ("Array of Strings 3")) -> (array=w558:string[])
    "?" <- w558
    n284 = Or(x=w483, y=w482) -> (x .or. y?=w481:bool)
    n285 = Or(x="Av-6Tt", y="DValve / AV6-T") -> (x .or. y?=w472:bool)
    n286 = Or(x="Reset Control", y="Reset FC") -> (x .or. y?=w507:bool)
    n287 = Or(x=w245, y=w231) -> (x .or. y?=w246:bool)
    n288 = local read "return"() -> (w486:bool)
    n289 = case shown="True" w472 {
      tunnel: [w726 w727] -> w475
      tunnel: w476 -> [w726 w728]
      frame False {
      }
      frame True {
        n290 = case shown="False" w728 {
          tunnel: [w730 _] -> w727
          frame False {
            w729 = TRUE
            n291 = local write "Control (on/off)"(w729) -> ()
            n292 = local write "av6-t ind"(w729) -> ()
            n293 = local read "Control input"() -> (w730:bool)
          }
          frame True {
            w731 = FALSE
            n294 = local write "Av-6Tt"(w731) -> ()
            n295 = local write "DValve / AV6-T"(w731) -> ()
          }
        }
      }
    }
    "AV6-T" <- w475
    "?" <- w475
    n296 = case shown="True" w231 {
      tunnel: [_ "o" ("write buffer")] -> w178
      tunnel: w505 -> [w768 w778]
      tunnel: [w769 w774] -> w506
      tunnel: w507 -> [w767 _]
      frame False {
        n297 = case shown="False" w767 {
          tunnel: [w770 200.0] -> w769
          tunnel: w768 -> [w770 _]
          frame False {
          }
          frame True {
          }
        }
        n298 = property on="Profile Selector" class="DigNum (strict)"("DisabledEnum"=0) -> ()  [unwired: 2 in, 2 out]
      }
      frame True {
        # "Send 'o' Takeoff"
        n299 = Subtract(x=w778, y=0.0) -> (x-y=w775:dbl)
        n300 = Greater Than 0?(x=w775) -> (x > 0?=w776:bool)
        n301 = case shown="False" w776 {
          selector: w776 -> [_ w783]
          tunnel: w775 -> [_ w784]
          tunnel: [w779 w784] -> w774
          frame False {
            n302 = local read "Takeoff Started"() -> (w780:bool)
            n303 = case shown="False" w780 {
              tunnel: [200.0 0.0] -> w779
              frame False {
              }
              frame True {
              }
            }
          }
          frame True {
            "Takeoff Started" <- w783
          }
        }
        n304 = property on="Profile Selector" class="DigNum (strict)"("DisabledEnum"=2) -> ()  [unwired: 2 in, 2 out]
      }
    }
    "?" <- w506
    n305 = Or(x=w246, y=w481) -> (x .or. y?=w484:bool)
    n306 = Array Size(array=w558) -> (size(s)=w559:i32)
    n307 = for {
      N: w559 -> [_]
      tunnel: w558 -> [w824]
      tunnel: [w816] -> w504 mode=concatenating
      i -> [w823]
      n308 = Index Array(array=w824, index=w823) -> (element=w819:string)
      n309 = String Subset(string=w819, offset (0)=2) -> (substring=w817:string)  [unwired: 1 in]
      n310 = Spreadsheet String To Array(delimiter (Tab)=",", format string="%d", spreadsheet string=w817, array type (2D Dbl)=string[] ["p:1234.1234.1234.1234,1234,1234", "t:1234,1234,1234"] ("Array of Strings 3")) -> (array=w816:string[])
    }
    n311 = Or(x=w486, y=w484) -> (x .or. y?=w487:bool)
    n312 = And(x=w486, y=w487) -> (x .and. y?=w485:bool)
    n313 = case shown="True" w485 {
      tunnel: w231 -> [_ w689]
      tunnel: w468 -> [_ w692]
      tunnel: w467 -> [_ w691]
      tunnel: [_ w690] -> _
      tunnel: w249 -> [_ w690]
      tunnel: w466 -> [_ w688]
      tunnel: w245 -> [_ w686]
      tunnel: w242 -> [_ w685]
      tunnel: w239 -> [_ w682]
      frame False {
      }
      frame True {
        n314 = local read "fc-u"() -> (w683:bool)
        n315 = case shown="True" w689 {
          frame False {
            w724 = FALSE
            n316 = local write "return"(w724) -> ()
            n317 = local write "Control (on/off)"(w724) -> ()
            n318 = local write "Control input"(w724) -> ()
          }
          frame True {
            w725 = FALSE
            n319 = local write "return"(w725) -> ()
            n320 = local write "Control (on/off)"(w725) -> ()
            n321 = local write "Control input"(w725) -> ()
          }
        }
        n322 = case shown="True" w683 {
          tunnel: w682 -> [_ w699]
          frame False {
          }
          frame True {
            n323 = local write "fc-u"(FALSE) -> ()
            n324 = case shown="True" w699 {
              frame False {
                n325 = local write "FC-U Toggle"(FALSE) -> ()
              }
              frame True {
                n326 = local write "FC-U Toggle"(FALSE) -> ()
              }
            }
          }
        }
        n327 = local read "soft kill ind"() -> (w697:bool)
        n328 = local read "abort ind"() -> (w694:bool)
        n329 = local read "av6-t ind"() -> (w693:bool)
        n330 = local read "run ind"() -> (w695:bool)
        n331 = local read "dump fuel ind"() -> (w696:bool)
        n332 = local read "fo-u"() -> (w687:bool)
        n333 = case shown="True" w694 {
          tunnel: w688 -> [_ w716]
          frame False {
          }
          frame True {
            n334 = local write "abort"(w716) -> ()
            n335 = local write "abort ind"(FALSE) -> ()
          }
        }
        n336 = case shown="True" w697 {
          tunnel: w689 -> [_ _]
          tunnel: w692 -> [_ w718]
          frame False {
          }
          frame True {
            n337 = local write "Soft Kill"(w718) -> ()
            n338 = local write "soft kill ind"(FALSE) -> ()
          }
        }
        n339 = case shown="True" w695 {
          tunnel: w689 -> [_ w723]
          frame False {
          }
          frame True {
            n340 = local write "Takeoff"(w723) -> ()
            n341 = local write "Test Run"(w723) -> ()
            n342 = local write "run ind"(FALSE) -> ()
          }
        }
        n343 = case shown="True" w693 {
          tunnel: w691 -> [_ w711]
          frame False {
          }
          frame True {
            n344 = case shown="True" w711 {
              frame False {
                n345 = local write "Av-6Tt"(FALSE) -> ()
                n346 = local write "DValve / AV6-T"(FALSE) -> ()
              }
              frame True {
                n347 = local write "Av-6Tt"(FALSE) -> ()
                n348 = local write "DValve / AV6-T"(FALSE) -> ()
              }
            }
            n349 = local write "av6-t ind"(FALSE) -> ()
          }
        }
        n350 = case shown="True" w696 {
          tunnel: w690 -> [_ w720]
          frame False {
          }
          frame True {
            n351 = local write "dump fuel"(w720) -> ()
            n352 = local write "dump fuel ind"(FALSE) -> ()
          }
        }
        n353 = case shown="True" w687 {
          tunnel: w686 -> [_ w706]
          frame False {
          }
          frame True {
            n354 = case shown="True" w706 {
              frame False {
                n355 = local write "FOU"(FALSE) -> ()
              }
              frame True {
                n356 = local write "FOU"(FALSE) -> ()
              }
            }
            n357 = local write "fo-u"(FALSE) -> ()
          }
        }
        n358 = local read "av5-m"() -> (w684:bool)
        n359 = case shown="True" w684 {
          tunnel: w685 -> [_ w702]
          frame False {
          }
          frame True {
            n360 = case shown="False" w702 {
              frame False {
                n361 = local write "tank iso"(FALSE) -> ()
              }
              frame True {
                n362 = local write "tank iso"(FALSE) -> ()
              }
            }
            n363 = local write "av5-m"(FALSE) -> ()
          }
        }
      }
    }
    n364 = Not(x="Primary Safety") -> ()  [unwired: 1 out]
    n365 = case shown="False" "Primary Safety" {
      tunnel: [0 2] -> w325
      tunnel: [w672 FALSE] -> w323
      frame False {
        n366 = property on="Full Power" class="Bool (strict)"() -> ("Value"=w672:bool)  [unwired: 2 in, 2 out]
      }
      frame True {
      }
    }
    n367 = Not(x="Primary Safety") -> (.not. x?=w331:bool)
    n368 = case shown="False" "Simulate" {
      tunnel: w504 -> [w754 w755]
      tunnel: [w754 w755] -> w409
      tunnel: [_ w755] -> w503
      frame False {
      }
      frame True {
      }
    }
    "?" <- w409
    n369 = case shown="True" "PixHawk" {
      tunnel: [_ "y" ("write buffer")] -> w526
      frame False {
      }
      frame True {
        # "Send 'y' Turn on Pixhawk"
      }
    }
    n370 = case shown="True" w331 {
      tunnel: [_ "s" ("write buffer")] -> w530
      frame False {
      }
      frame True {
        # "Send 's' to disengage safety"
      }
    }
    n371 = case shown="True" w507 {
      tunnel: [_ "r" ("write buffer")] -> w528
      frame False {
      }
      frame True {
        # "Send 'r' Reset Flight Computer"
      }
    }
    n372 = case shown="True" "Simulate" {
      tunnel: [_ "p" ("write buffer")] -> w525
      frame False {
      }
      frame True {
        # "Send 'p' begin flight profile sim"
        n373 = property on="Profile Selector" class="DigNum (strict)"("DisabledEnum"=2) -> ()  [unwired: 2 in, 2 out]
      }
    }
    n374 = Or(x="Flight Control Board", y="Full Power") -> (x .or. y?=w517:bool)
    n375 = case shown="True" w245 {
      tunnel: [_ "d"] -> w516
      frame False {
      }
      frame True {
      }
    }
    n376 = case shown="True" "Simulate" {
      tunnel: [_ w562] -> w176
      frame False {
      }
      frame True {
        n377 = property on="Profile Selector" class="DigNum (strict)"() -> ("Value"=w563:u16)  [unwired: 2 in, 2 out]
        n378 = Format Into String(w563) -> (resulting string=w562:string)  [unwired: 3 in, 1 out]
      }
    }
    n379 = case shown="True" w517 {
      tunnel: [_ "z" ("write buffer")] -> w529
      frame False {
      }
      frame True {
        # "Send 'z' Turn on Power"
      }
    }
    n380 = case shown="True" w249 {
      tunnel: [_ "b" ("write buffer")] -> w512
      frame False {
      }
      frame True {
        # "Send 'b' Dump FUEL"
      }
    }
    n381 = case shown="True" w475 {
      tunnel: [_ "v" ("write buffer")] -> w513
      frame False {
      }
      frame True {
        # "Send 'v' Dump Valve"
      }
    }
    n382 = property on="Full Power" class="Bool (strict)"("Value"=w323) -> ()  [unwired: 2 in, 2 out]
    n383 = property on="Full Power" class="Bool (strict)"("DisabledEnum"=w325) -> ()  [unwired: 2 in, 2 out]
    n384 = property on="Takeoff" class="Bool (strict)"() -> ("Value"=w174:bool)  [unwired: 2 in, 2 out]
    n385 = case shown="True" w174 {
      tunnel: [_ w564] -> w177
      frame False {
      }
      frame True {
        n386 = property on="Profile Selector" class="DigNum (strict)"() -> ("Value"=w565:u16)  [unwired: 2 in, 2 out]
        n387 = Format Into String(w565) -> (resulting string=w564:string)  [unwired: 3 in, 1 out]
      }
    }
    n388 = case shown="True" w239 {
      tunnel: [_ "i"] -> w515
      frame False {
      }
      frame True {
        (unwired) TRUE
      }
    }
    n389 = case shown="True" w242 {
      tunnel: [_ "t"] -> w514
      frame False {
      }
      frame True {
      }
    }
    n390 = case shown="True" w466 {
      tunnel: [_ "a" ("write buffer")] -> w511
      frame False {
      }
      frame True {
        # "Send 'a' ABORT"
        n391 = property on="Secondary Safety" class="Bool (strict)"("Value"=TRUE) -> ()  [unwired: 2 in, 2 out]
      }
    }
    n392 = case shown="True" w468 {
      tunnel: [_ "k" ("write buffer")] -> w527
      frame False {
      }
      frame True {
        # "Send 'k' softkill"
      }
    }
    n393 = case shown="True" "Fan Shutdown" {
      tunnel: [_ "f"] -> w232
      frame False {
      }
      frame True {
        # "Sends 'f' to shut off fan"
      }
    }
    n394 = Array Size(array=w409) -> (size(s)=w408:i32)
    n395 = Index Array(array=w503, index=0) -> (element=w502:string)
    "String" <- w502
    n396 = Index Array(array=w409, index=0) -> (element=w551:string)
    n397 = Index Array(array=w409, index=7) -> (element=w540:string)
    n398 = Index Array(array=w409, index=1) -> (element=w550:string)
    n399 = Index Array(array=w409, index=8) -> (element=w539:string)
    n400 = Index Array(array=w409, index=2) -> (element=w549:string)
    n401 = Index Array(array=w409, index=9) -> (element=w538:string)
    n402 = Index Array(array=w409, index=3) -> (element=w548:string)
    n403 = Index Array(array=w409, index=4) -> (element=w547:string)
    n404 = Index Array(array=w409, index=5) -> (element=w546:string)
    n405 = Index Array(array=w409, index=6) -> (element=w509:string)
    n406 = Index Array(array=w409, index=13) -> (element=w531:string)
    n407 = Index Array(array=w409, index=10) -> (element=w536:string)
    n408 = Index Array(array=w409, index=11) -> (element=w535:string)
    n409 = Index Array(array=w409, index=12) -> (element=w534:string)
    n410 = Index Array(array=w409, index=16) -> (element=w451:string)
    n411 = Index Array(array=w409, index=14) -> (element=w453:string)
    n412 = Index Array(array=w409, index=15) -> (element=w452:string)
    n413 = Index Array(array=w409, index=17) -> (element=w450:string)
    n414 = Fract/Exp String To Number(string=w551) -> (number=w348:dbl)  [unwired: 3 in, 1 out]
    n415 = Fract/Exp String To Number(string=w550) -> (number=w347:dbl)  [unwired: 3 in, 1 out]
    n416 = Fract/Exp String To Number(string=w549) -> (number=w346:dbl)  [unwired: 3 in, 1 out]
    n417 = Fract/Exp String To Number(string=w548) -> (number=w345:dbl)  [unwired: 3 in, 1 out]
    n418 = Fract/Exp String To Number(string=w531) -> (number=w298:dbl)  [unwired: 3 in, 1 out]
    n419 = Fract/Exp String To Number(string=w547) -> (number=w344:dbl)  [unwired: 3 in, 1 out]
    n420 = Fract/Exp String To Number(string=w546) -> (number=w343:dbl)  [unwired: 3 in, 1 out]
    n421 = Fract/Exp String To Number(string=w509) -> (number=w342:dbl)  [unwired: 3 in, 1 out]
    n422 = Fract/Exp String To Number(string=w451) -> (number=w255:dbl)  [unwired: 3 in, 1 out]
    n423 = Fract/Exp String To Number(string=w453) -> (number=w269:dbl)  [unwired: 3 in, 1 out]
    n424 = Fract/Exp String To Number(string=w452) -> (number=w264:dbl)  [unwired: 3 in, 1 out]
    n425 = Fract/Exp String To Number(string=w450) -> (number=w250:dbl)  [unwired: 3 in, 1 out]
    n426 = Decrement(x=w408) -> (x-1=w407:i32)
    n427 = Fract/Exp String To Number(string=w540) -> (number=w297:dbl)  [unwired: 3 in, 1 out]
    "TCpw-1" <- w297
    n428 = Fract/Exp String To Number(string=w539) -> (number=w296:dbl)  [unwired: 3 in, 1 out]
    "TCpw-2" <- w296
    n429 = Fract/Exp String To Number(string=w538) -> (number=w295:dbl)  [unwired: 3 in, 1 out]
    "TCpw-3" <- w295
    n430 = Fract/Exp String To Number(string=w536) -> (number=w294:dbl)  [unwired: 3 in, 1 out]
    "TCpw-4" <- w294
    n431 = Fract/Exp String To Number(string=w535) -> (number=w291:dbl)  [unwired: 3 in, 1 out]
    "TCp-1" <- w291
    n432 = Fract/Exp String To Number(string=w534) -> (number=w290:dbl)  [unwired: 3 in, 1 out]
    "TCp-2" <- w290
    n433 = local read "Multiplier 1"() -> (w374:dbl)
    n434 = local read "Multiplier 2"() -> (w372:dbl)
    n435 = local read "Multiplier 3"() -> (w370:dbl)
    n436 = local read "Multiplier 4"() -> (w368:dbl)
    n437 = local read "Multiplier 5"() -> (w366:dbl)
    n438 = local read "Multiplier 6"() -> (w363:dbl)
    n439 = Equal?(x=w502, y="String 3") -> (x = y?=→"?":bool)
    n440 = Index Array(array=w409, index=w407) -> (element=w412:string)
    n441 = Concatenate Strings("h" ("string"), ":" ("string"), w530, w529, w528, w516, w526, w525, w232, w527, w515, w514, w513, w511, w512, w176, w177, w178, ";" ("string")) -> (w458:string)
    "Output" <- w458
    n442 = Divide(x=w269, y=10.0) -> (x/y=w267:dbl)
    n443 = Divide(x=w264, y=10.0) -> (x/y=w260:dbl)
    n444 = Divide(x=w255, y=10.0) -> (x/y=w257:dbl)
    n445 = Divide(x=w250, y=10.0) -> (x/y=w252:dbl)
    n446 = local read "Multiplier 7"() -> (w361:dbl)
    n447 = Subtract(x=w267, y=100.0) -> (x-y=→"Engine 1":dbl)
    n448 = Subtract(x=w257, y=100.0) -> (x-y=→"Engine 3":dbl)
    n449 = Subtract(x=w252, y=100.0) -> (x-y=→"Engine 4":dbl)
    n450 = Multiply(x=w348, y=w374) -> (x*y=w381:dbl)
    n451 = Multiply(x=w347, y=w372) -> (x*y=w380:dbl)
    n452 = Multiply(x=w346, y=w370) -> (x*y=w379:dbl)
    n453 = Multiply(x=w345, y=w368) -> (x*y=w378:dbl)
    n454 = Multiply(x=w344, y=w366) -> (x*y=w377:dbl)
    n455 = Multiply(x=w343, y=w363) -> (x*y=w376:dbl)
    n456 = Subtract(x=w260, y=100.0) -> (x-y=→"Engine 2":dbl)
    n457 = Bundle(w269, w264, w255, w250) -> (→"Motors":cluster{dbl, dbl, dbl, dbl})  [unwired: 1 in]
    n458 = Equal?(x=w297, y=-1.0) -> (x = y?=→"TCpw-1":bool)
    n459 = Equal?(x=w297, y=-3.0) -> (x = y?=→"vcc":bool)
    n460 = Equal?(x=w297, y=-2.0) -> (x = y?=→"gnd":bool)
    n461 = Equal?(x=w296, y=-2.0) -> (x = y?=→"gnd 2":bool)
    n462 = Equal?(x=w296, y=-3.0) -> (x = y?=→"vcc 2":bool)
    n463 = Equal?(x=w296, y=-1.0) -> (x = y?=→"TCpw-2":bool)
    n464 = Equal?(x=w295, y=-3.0) -> (x = y?=→"vcc 3":bool)
    n465 = Equal?(x=w295, y=-2.0) -> (x = y?=→"gnd 3":bool)
    n466 = Equal?(x=w295, y=-1.0) -> (x = y?=→"TCpw-3":bool)
    n467 = Equal?(x=w294, y=-2.0) -> (x = y?=→"gnd 4":bool)
    n468 = Equal?(x=w294, y=-1.0) -> (x = y?=→"TCpw-4":bool)
    n469 = Equal?(x=w294, y=-3.0) -> (x = y?=→"vcc 4":bool)
    n470 = Equal?(x=w291, y=-3.0) -> (x = y?=→"vcc 5":bool)
    n471 = Equal?(x=w291, y=-2.0) -> (x = y?=→"gnd 5":bool)
    n472 = Equal?(x=w291, y=-1.0) -> (x = y?=→"TCp-1":bool)
    n473 = Equal?(x=w290, y=-3.0) -> (x = y?=→"vcc 6":bool)
    n474 = Equal?(x=w290, y=-1.0) -> (x = y?=→"TCp-2":bool)
    n475 = Equal?(x=w290, y=-2.0) -> (x = y?=→"gnd 6":bool)
    n476 = Index Array(array=w409, index=18) -> (element=w352:string)
    n477 = Fract/Exp String To Number(string=w412) -> (number=→"ms":dbl)  [unwired: 3 in, 1 out]
    n478 = Equal?(x=w458, y=w352) -> (x = y?=w460:bool)
    n479 = Multiply(x=w342, y=w361) -> (x*y=w375:dbl)
    n480 = Search/Split String(string=w352, search string/char (-)="r") -> (offset of match=w398:i32)  [unwired: 1 in, 2 out]
    n481 = Search/Split String(string=w352, search string/char (-)="z") -> (offset of match=w400:i32)  [unwired: 1 in, 2 out]
    n482 = Search/Split String(string=w352, search string/char (-)="s") -> (offset of match=w402:i32)  [unwired: 1 in, 2 out]
    n483 = Search/Split String(string=w352, search string/char (-)="k") -> (offset of match=w464:i32)  [unwired: 1 in, 2 out]
    n484 = Search/Split String(string=w352, search string/char (-)="a") -> (offset of match=w405:i32)  [unwired: 1 in, 2 out]
    n485 = Search/Split String(string=w352, search string/char (-)="t") -> (offset of match=w394:i32)  [unwired: 1 in, 2 out]
    n486 = case shown="False" w460 {
      tunnel: [w681 _] -> w459
      tunnel: w458 -> [w681 _]
      frame False {
      }
      frame True {
      }
    }
    n487 = local read "Offset 1"() -> (w373:dbl)
    n488 = local read "Offset 2"() -> (w371:dbl)
    n489 = local read "Offset 3"() -> (w369:dbl)
    n490 = local read "Offset 4"() -> (w367:dbl)
    n491 = local read "Offset 5"() -> (w365:dbl)
    n492 = local read "Offset 6"() -> (w364:dbl)
    n493 = local read "Offset 7"() -> (w362:dbl)
    n494 = Greater Or Equal To 0?(x=w464) -> (x >= 0?=→"Craft Triggered Softkill Active":bool)
    n495 = Greater Or Equal To 0?(x=w405) -> (x >= 0?=w332:bool)
    "Hardkill Active" <- w332
    n496 = Greater Or Equal To 0?(x=w398) -> (x >= 0?=w337:bool)
    "Reset Triggered" <- w337
    n497 = Greater Or Equal To 0?(x=w400) -> (x >= 0?=w360:bool)
    "Flight Control On" <- w360
    n498 = Greater Or Equal To 0?(x=w394) -> (x >= 0?=w389:bool)
    n499 = Greater Or Equal To 0?(x=w402) -> (x >= 0?=w390:bool)
    "Primary Safety Active" <- w390
    n500 = Multiply(x=0.0069, y=w298) -> (x*y=w209:dbl)
    n501 = Bundle(w297, w296, w295, w294) -> (→"?":cluster{dbl, dbl, dbl, dbl})  [unwired: 1 in]
    n502 = Bundle(w291, w290) -> (→"?":cluster{dbl, dbl})  [unwired: 1 in]
    n503 = local read "Manual Abort Tested"() -> (w395:bool)
    n504 = local read "Reset Triggered 2"() -> (w396:bool)
    n505 = Add(x=w373, y=w381) -> (x+y=w230:dbl)
    n506 = Add(x=w371, y=w380) -> (x+y=w227:dbl)
    n507 = Add(x=w369, y=w379) -> (x+y=w224:dbl)
    n508 = Add(x=w367, y=w378) -> (x+y=w221:dbl)
    n509 = Add(x=w365, y=w377) -> (x+y=w218:dbl)
    n510 = Add(x=w364, y=w376) -> (x+y=w215:dbl)
    n511 = Add(x=w362, y=w375) -> (x+y=w212:dbl)
    n512 = Add(x=11.144, y=w209) -> (x+y=w208:dbl)
    n513 = call "N_Point_Running_Average.vi"("n"=10, "Input"=w224) -> ("Output"=w223:dbl)
    "PT3-M" <- w223
    n514 = call "N_Point_Running_Average.vi"("n"=10, "Input"=w215) -> ("Output"=w214:dbl)
    "PT2-M" <- w214
    n515 = call "N_Point_Running_Average.vi"("n"=10, "Input"=w212) -> ("Output"=w211:dbl)
    "PT5-M" <- w211
    n516 = call "N_Point_Running_Average.vi"("n"=10, "Input"=w221) -> ("Output"=w220:dbl)
    "PT1-U" <- w220
    n517 = call "N_Point_Running_Average.vi"("n"=10, "Input"=w218) -> ("Output"=w217:dbl)
    "PT2-U" <- w217
    n518 = call "N_Point_Running_Average.vi"("n"=5, "Input"=w208) -> ("Output"=w173:dbl)
    "Voltage Sensor" <- w173
    "?" <- w173
    n519 = call "N_Point_Running_Average.vi"("n"=10, "Input"=w227) -> ("Output"=w226:dbl)
    "PT1-M" <- w226
    n520 = call "N_Point_Running_Average.vi"("n"=10, "Input"=w230) -> ("Output"=w229:dbl)
    "PT4-M" <- w229
    n521 = Or(x=w395, y=w332) -> (x .or. y?=w392:bool)
    "Manual Abort Tested" <- w392
    n522 = Or(x=w396, y=w337) -> (x .or. y?=w391:bool)
    "Reset Triggered 2" <- w391
    n523 = property on="Craft Triggered Softkill Active" class="Bool (strict)"() -> ("Value"=w185:bool)  [unwired: 2 in, 2 out]
    n524 = property on="Hardkill Active" class="Bool (strict)"() -> ("Value"=w184:bool)  [unwired: 2 in, 2 out]
    n525 = Build Array(w348, w347, w346, w345, w344, w343, w342, w229, w226, w223, w220, w217, w214, w211, w297, w296, w295, w294, w291, w290, w173, w269, w264, w264, w250) -> (w355:dbl[])
    n526 = Bundle("Output"=w173, w297, w296, w295, w294, w291, w290, "Output"=w229, "Output"=w226, "Output"=w223, "Output"=w220, "Output"=w217, "Output"=w214, "Output"=w211) -> (w339:T5)  [unwired: 1 out]
    n527 = property on="PT1-U" class="DigNum (strict)"() -> ("Value"=w181:dbl)  [unwired: 2 in, 2 out]
    n528 = Or(x=w185, y=w184) -> (x .or. y?=w183:bool)
    n529 = Greater?(x=w181, y=4900.0) -> (0:→"PT1-U > 4900 PSI":bool)
    n530 = Bundle("Output"=w220, "Output"=w217) -> (→"?":cluster{"Output":dbl, "Output":dbl})  [unwired: 1 in]
    n531 = Build Array(w392, w391, w360, w389, w390) -> (w388:bool[])
    n532 = Bundle("Output"=w226, "Output"=w214, "Output"=w223, "Output"=w229, "Output"=w211) -> (→"?":T6)  [unwired: 1 in]
    n533 = case shown="True" "Send" {
      tunnel: w406 -> [_ w791]
      tunnel: w459 -> [_ w790]
      tunnel: w338 -> [_ w789]
      frame False {
      }
      frame True {
        n534 = case shown="No Error" w791 {
          selector: w791 -> [w794 w798]
          tunnel: [w796 w797] -> _
          tunnel: [w795 w798] -> _
          tunnel: w790 -> [w793 _]
          tunnel: w789 -> [w792 w797]
          frame No Error {
            n535 = VISA Write(VISA resource name=w792, write buffer=w793, error in (no error)=w794) -> (VISA resource name out=w796:refnum<visa-resource-name>, error out=w795:errorcluster)  [unwired: 1 out]
          }
          frame Error {
          }
        }
      }
    }
    n536 = case shown="True" w183 {
      frame False {
        w566 = 0
        n537 = property on="AV1-T" class="Bool (strict)"("DisabledEnum"=w566) -> ()  [unwired: 2 in, 2 out]
        n538 = property on="AV5-T" class="Bool (strict)"("DisabledEnum"=w566) -> ()  [unwired: 2 in, 2 out]
        n539 = property on="AV4-T" class="Bool (strict)"("DisabledEnum"=w566) -> ()  [unwired: 2 in, 2 out]
        n540 = property on="AV2-T" class="Bool (strict)"("DisabledEnum"=w566) -> ()  [unwired: 2 in, 2 out]
        n541 = property on="AV3-T" class="Bool (strict)"("DisabledEnum"=w566) -> ()  [unwired: 2 in, 2 out]
        n542 = property on="FO-U" class="Bool (strict)"("DisabledEnum"=w566) -> ()  [unwired: 2 in, 2 out]
        n543 = property on="FC-U" class="Bool (strict)"("DisabledEnum"=w566) -> ()  [unwired: 2 in, 2 out]
        n544 = property on="AV6-T" class="Bool (strict)"("DisabledEnum"=w566) -> ()  [unwired: 2 in, 2 out]
      }
      frame True {
        w567 = 2
        n545 = property on="FC-U" class="Bool (strict)"("DisabledEnum"=w567) -> ()  [unwired: 2 in, 2 out]
        n546 = property on="AV5-T" class="Bool (strict)"("DisabledEnum"=w567) -> ()  [unwired: 2 in, 2 out]
        n547 = property on="AV4-T" class="Bool (strict)"("DisabledEnum"=w567) -> ()  [unwired: 2 in, 2 out]
        n548 = property on="AV3-T" class="Bool (strict)"("DisabledEnum"=w567) -> ()  [unwired: 2 in, 2 out]
        n549 = property on="AV2-T" class="Bool (strict)"("DisabledEnum"=w567) -> ()  [unwired: 2 in, 2 out]
        n550 = property on="AV6-T" class="Bool (strict)"("DisabledEnum"=w567) -> ()  [unwired: 2 in, 2 out]
        n551 = property on="AV1-T" class="Bool (strict)"("DisabledEnum"=w567) -> ()  [unwired: 2 in, 2 out]
        n552 = property on="FO-U" class="Bool (strict)"("DisabledEnum"=w567) -> ()  [unwired: 2 in, 2 out]
      }
    }
    n553 = Array To Spreadsheet String(delimiter (Tab)="\t", array=w355, 3:"%f" ("format string")) -> (spreadsheet string=w336:string)
    n554 = Max & Min(x=w340, y=w339) -> (max(x,y)=w341:T3)  [unwired: 1 out]
    "Max Values" <- w341
    n555 = And Array Elements(Boolean array=w388) -> (logical AND=w384:bool)
    n556 = Search/Split String(string=w336, search string/char (-)="\r\n") -> (substring before match=w334:string)  [unwired: 1 in, 2 out]
    n557 = And(x=w387, y=w384) -> (x .and. y?=w386:bool)
    n558 = Concatenate Strings(w334, "\t" ("string"), w352, "\n" ("string")) -> (w350:string)
    n559 = Or(x=w387, y=w386) -> (x .or. y?=w385:bool)
    n560 = Write to Text File(file (use dialog)=w359, text=w350) -> (refnum out=w356:refnum<file>)  [unwired: 2 in, 2 out]
    n561 = Exclusive Or(1:w385, 2:"Begin Checklist") -> (0:w403:bool)
    n562 = case shown="True" w403 {
      frame False {
      }
      frame True {
        w680 = FALSE
        n563 = local write "Reset Triggered 2"(w680) -> ()
        n564 = local write "Manual Abort Tested"(w680) -> ()
      }
    }
    n565 = Wait Until Next ms Multiple(millisecond multiple=200) -> ()  [unwired: 1 out]
    "Iterations" <- w326
  }
  n566 = VISA Open(VISA resource name=refnum<visa-resource-name> "COM3") -> (VISA resource name=w5:refnum<visa-resource-name>, error out=w4:errorcluster)  [unwired: 4 in]
  n567 = VISA Close(VISA resource name=w5, error in (no error)=w4) -> ()  [unwired: 1 out]
  n568 = VISA Close(VISA resource name=w7, error in (no error)=w61) -> ()  [unwired: 1 out]
  n569 = Close File(refnum=w58) -> ()  [unwired: 1 in, 2 out]
